vi "ternaryoprator.vi"() -> ()   [LabVIEW 2019]
panel:
  out "var":string
  in  "iinput":dbl
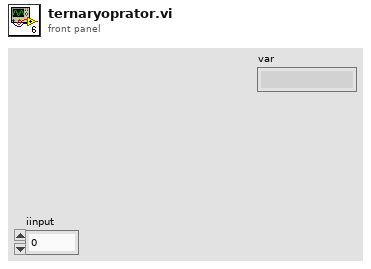
[diagram p1: front panel]
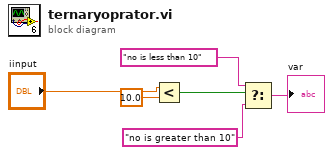
[diagram p0: block diagram]
diagram:
  n1 = Less?(x="iinput", y=10.0) -> (x < y?=w4:bool)
  n2 = Select(t="no is less than 10", s=w4, f="no is greater than 10") -> (s? t:f=→"var":string)
